vi "set_lock.vi"(6 "error in (no error)":errorcluster, 7 "lock cell":bool, 8 "heat_board_control in":refnum<class "heat_board_control.lvclass">) -> (0 "error out":errorcluster, 5 "heat_board_control out":refnum<class "heat_board_control.lvclass">)   [LabVIEW 2015, in "heat_board_control.lvclass"]
uses:
  heat_board_control.lvclass
  heat_board_control.lvclass/heat_board_control.ctl
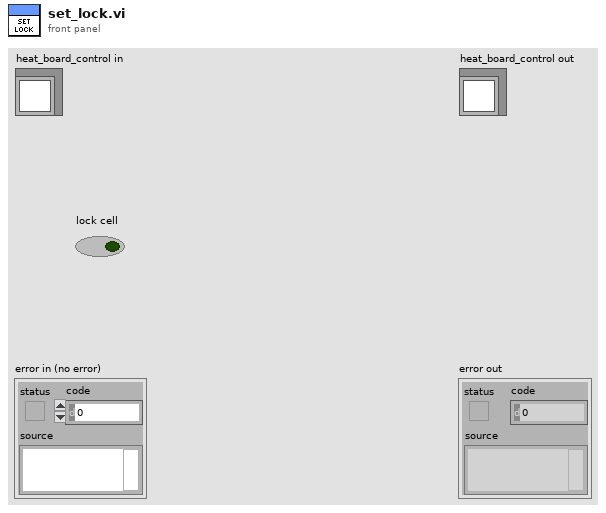
[diagram p1: front panel]
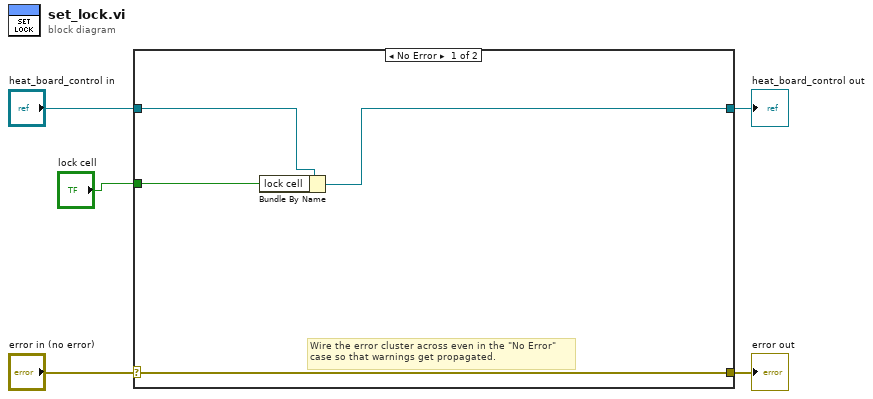
[diagram p0: block diagram]
diagram:
  n1 = case shown="No Error" "error in (no error)" {
    selector: "error in (no error)" -> [w9 w11]
    tunnel: [w9 w11] -> w4
    tunnel: [w6 w10] -> w2
    tunnel: "heat_board_control in" -> [w7 w10]
    tunnel: "lock cell" -> [w8 _]
    frame No Error {
      # "Wire the error cluster across even in the \"No Error\"\ncase so that warnings get propagated."
      n2 = Bundle By Name(cluster=w7, "lock cell"=w8) -> (w6:refnum<class "heat_board_control.lvclass">)
    }
    frame Error {
    }
  }
  "error out" <- w4
  "heat_board_control out" <- w2
